vi "SBOM JSON Probe.vi"(11 "CycloneDX SBOM out":refnum<class "CycloneDX JSON.lvclass">) -> (2 "Value String":string, 3 "Boolean":bool)   [LabVIEW 2017, in "LabVIEW CycloneDX SBOM.lvlib" / "CycloneDX JSON.lvclass"]
uses:
  CycloneDX JSON.lvclass
  <vilib>/JDP Science/JSONtext/JSONtext.lvlib
panel:
  out "Value String 2":string
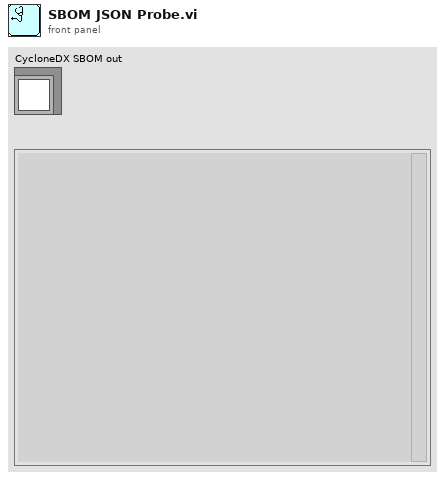
[diagram p1: front panel]
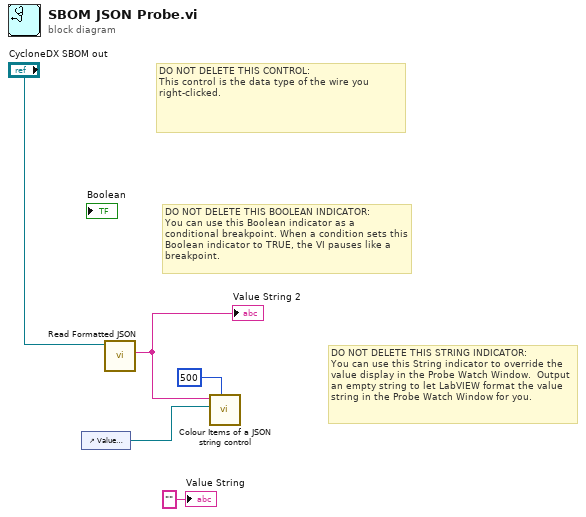
[diagram p0: block diagram]
diagram:
  # "DO NOT DELETE THIS STRING INDICATOR: \nYou can use this String indicator to override the value display in the Probe Watch Window.  Output an empty string to let LabVIEW format the value string in the Probe Watch Window for you."
  # "DO NOT DELETE THIS BOOLEAN INDICATOR: \nYou can use this Boolean indicator as a conditional breakpoint. When a condition sets this Boolean indicator to TRUE, the VI pauses like a breakpoint."
  # "DO NOT DELETE THIS CONTROL: \nThis control is the data type of the wire you right-clicked."
  n1 = control-ref of="Value String 2"() -> (w2:refnum<vi>)
  n2 = call "Read Formatted JSON.vi"("CycloneDX SBOM in"="CycloneDX SBOM out") -> ("JSON"=w3:string)  [unwired: 8 in, 2 out]
  "Value String 2" <- w3
  n3 = call <vilib>:"Colour Items of a JSON string control.vi"("Maximum UI Property calls"=500, "String Control"=w2, "JSON"=w3) -> ()  [unwired: 9 in]
  "Value String" <- "" ("Value String")
